vi "Configure Power Supply Rejection Ratio Analysis (Waveform).vi"(6 "Amplitude Range (1: F100Hz)":i32(ring)=1 items=["F20Hz", "F100Hz", "F1KHz", "F10KHz", "F100KHz", "F1MHz", "F10MHz", "F20MHz"], 7 "Impedance (1:50 Ohm)":i32(ring)=1 items=["1 MOhm", "50 Ohm"], 8 "error in (no error)":errorcluster, 9 "Amplitude (0.2)":dbl=0.2, 10 "Enable Initial Ramp Amplitude (F: Disable)":bool, 11 "VISA resource name":refnum<visa-resource-name>) -> (0 "error out":errorcluster, 3 "VISA resource name out":refnum<visa-resource-name>)   [LabVIEW 2015, in "Agilent 2000 3000 X-Series.lvlib"]
doc: "Configures the waveform generation parameters for power supply rejection ratio (PSRR) power analysis.\n\n<b>Note:</b>\n - This VI is applicable for 3000T,3000G, 4000, 6000 X-Series."
uses:
  Agilent 2000 3000 X-Series.lvlib
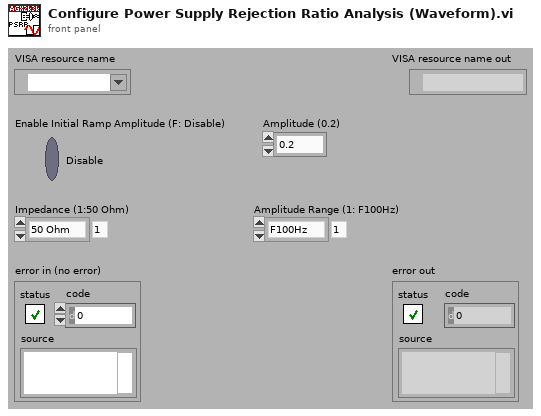
[diagram p1: front panel]
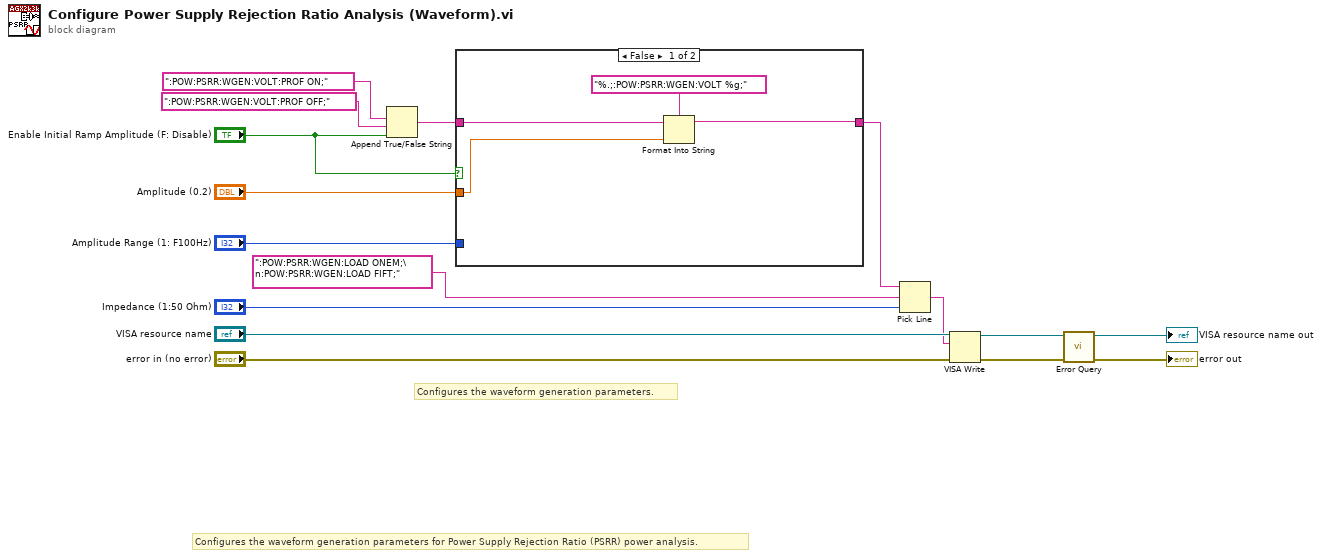
[diagram p0: block diagram]
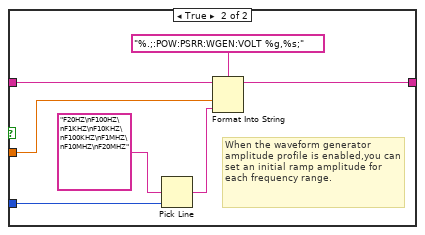
[diagram p2: hidden frame]
diagram:
  # "Configures the waveform generation parameters."
  # "Configures the waveform generation parameters for Power Supply Rejection Ratio (PSRR) power analysis."
  n1 = Append True/False String(1:"Enable Initial Ramp Amplitude (F: Disable)", 2:":POW:PSRR:WGEN:VOLT:PROF OFF;", 3:":POW:PSRR:WGEN:VOLT:PROF ON;") -> (0:w10:string)  [unwired: 1 in]
  n2 = case shown="False" "Enable Initial Ramp Amplitude (F: Disable)" {
    tunnel: w10 -> [w18 w24]
    tunnel: "Amplitude (0.2)" -> [w19 w23]
    tunnel: "Amplitude Range (1: F100Hz)" -> [_ w22]
    tunnel: [w17 w21] -> w6
    frame False {
      n3 = Format Into String(format string="%.;:POW:PSRR:WGEN:VOLT %g;", initial string=w18, w19) -> (resulting string=w17:string)  [unwired: 1 in, 1 out]
    }
    frame True {
      # "When the waveform generator amplitude profile is enabled,you can set an initial ramp amplitude for each frequency range."
      n4 = Pick Line(multi-line string="F20HZ\nF100HZ\nF1KHZ\nF10KHZ\nF100KHZ\nF1MHZ\nF10MHZ\nF20MHZ", line index=w22) -> (output string=w25:string)  [unwired: 1 in]
      n5 = Format Into String(format string="%.;:POW:PSRR:WGEN:VOLT %g,%s;", initial string=w24, w23, w25) -> (resulting string=w21:string)  [unwired: 1 in, 1 out]
    }
  }
  n6 = Pick Line(string ("")=w6, multi-line string=":POW:PSRR:WGEN:LOAD ONEM;\n:POW:PSRR:WGEN:LOAD FIFT;", line index="Impedance (1:50 Ohm)") -> (output string=w1:string)
  n7 = VISA Write(VISA resource name="VISA resource name", write buffer=w1, error in (no error)="error in (no error)") -> (VISA resource name out=w5:refnum<visa-resource-name>, error out=w4:errorcluster)  [unwired: 1 out]
  n8 = call "Error Query.vi"("error in (no error)"=w4, "VISA resource name"=w5) -> ("error out"=→"error out":errorcluster, "VISA resource name out"=→"VISA resource name out":refnum<visa-resource-name>)  [unwired: 6 in, 2 out]
